vi "Initialize.vi"(8 "error in (no error)":errorcluster, 10 "Internal?":bool, 11 "Huber Settings In":T1) -> (0 "error out":errorcluster, 2 "Connection Error":bool, 3 "Huber Settings Out":T1)   [LabVIEW 2018, in "Huber Unistat 410 TCU.lvlib"]
uses:
  Huber Unistat 410 TCU.lvlib
  Huber Unistat 410 Settings.ctl
  <vilib>/Instr/_visa.llb/VISA Configure Serial Port (Instr).vi
panel:
  out "read string":string
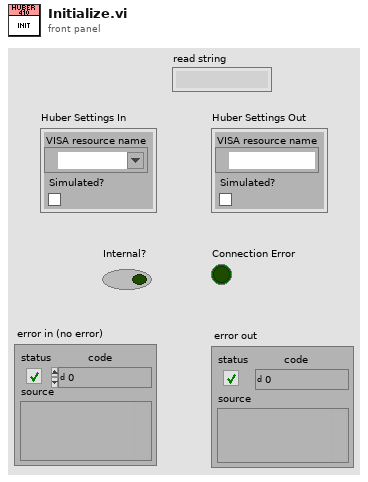
[diagram p1: front panel]
types:
  T1 = typedef "Huber Unistat 410 TCU.lvlib/Huber Unistat 410 Settings.ctl" = cluster{"VISA resource name":refnum<visa-resource-name>, "Simulated?":bool}
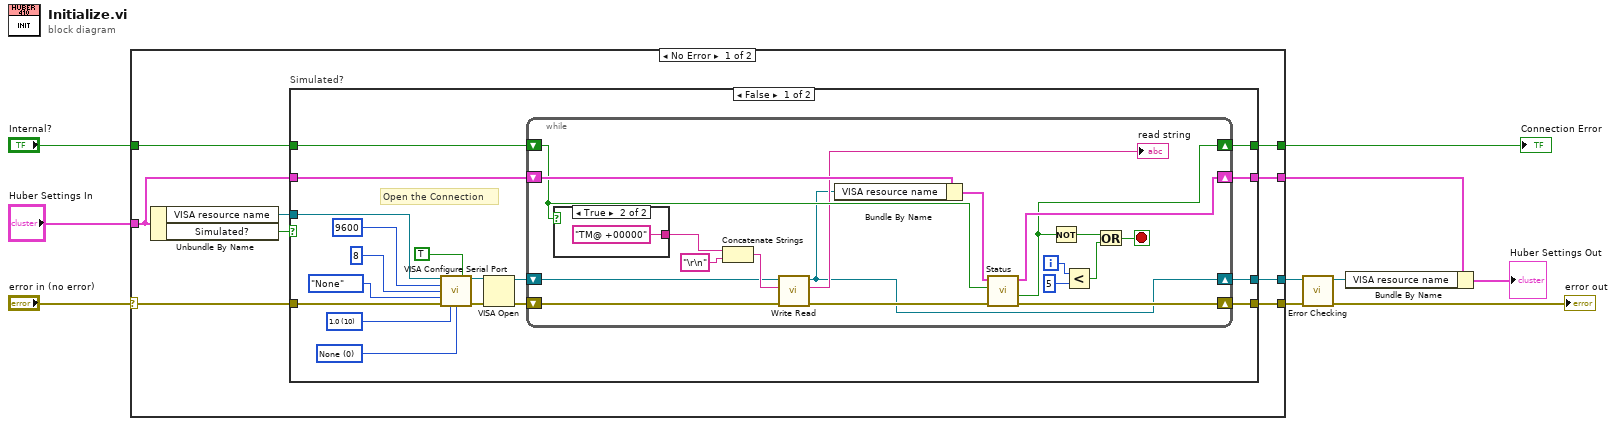
[diagram p0: block diagram]
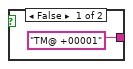
[diagram p2: hidden frame]
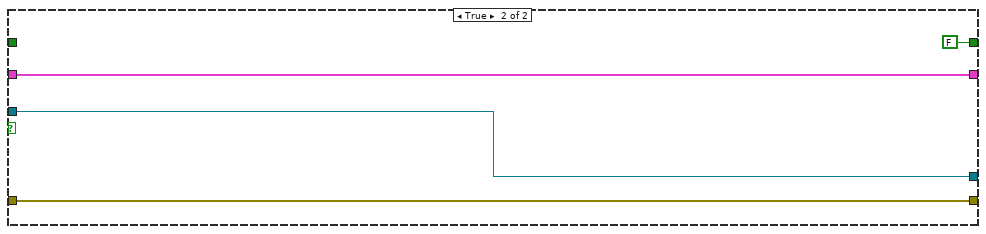
[diagram p3: hidden frame]
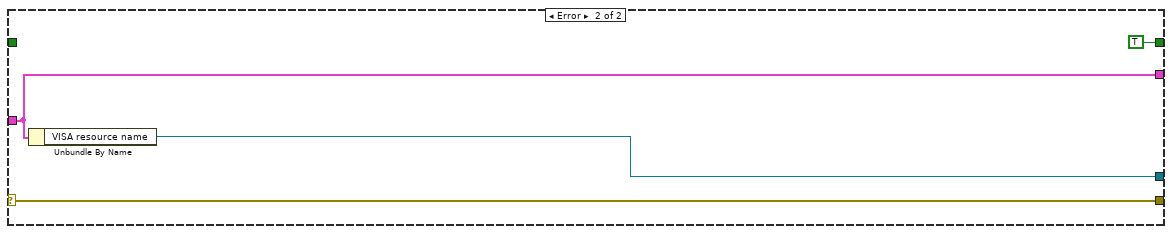
[diagram p4: hidden frame]
diagram:
  n1 = case shown="No Error" "error in (no error)" {
    selector: "error in (no error)" -> [w19 w66]
    tunnel: "Huber Settings In" -> [w13 w63]
    tunnel: [w18 w66] -> w8
    tunnel: [w16 w65] -> w9
    tunnel: [w14 TRUE] -> w4
    tunnel: [w12 w63] -> w3
    tunnel: "Internal?" -> [w11 _]
    frame No Error {
      n2 = Unbundle By Name(w13) -> ("VISA resource name"=w17:refnum<visa-resource-name>, "Simulated?"=w15:bool)
      n3 = case "Simulated?" shown="False" w15 {
        tunnel: w19 -> [w32 w62]
        tunnel: [w26 w62] -> w18
        tunnel: [w20 w61] -> w16
        tunnel: w17 -> [w31 w61]
        tunnel: [w28 FALSE] -> w14
        tunnel: w13 -> [w29 w59]
        tunnel: [w27 w59] -> w12
        tunnel: w11 -> [w25 _]
        frame False {
          w33 = u16 0 items=["None", "XON/XOFF", "RTS/CTS", "XON/XOFF & RTS/CTS", "DTR/DSR", "XON/XOFF & DTR/DSR"] ("flow control (0:none)")
          w34 = u16 10 items=["1.0"=10, "1.5"=15, "2.0"=20] ("stop bits (10: 1 bit)")
          # "Open the Connection"
          n4 = call-poly "VISA Configure Serial Port"("VISA resource name"=w31, "Enable Termination\nChar (T)"=TRUE ("Enable Termination\nChar (T)"), "baud rate (9600)"=u32 9600, "data bits (8)"=u16 8, "parity (0:none)"=enum16{"None", "Odd", "Even", "Mark", "Space"}."None", "error in (no error)"=w32, "stop bits (10: 1 bit)"=w34, "flow control (0:none)"=w33) -> ("VISA resource name out"=w23:refnum<visa-resource-name>, "error out"=w24:errorcluster)  [unwired: 6 in]
          n5 = VISA Open(error in (no error)=w24, VISA resource name=w23) -> (VISA resource name=w21:refnum<visa-resource-name>, error out=w22:errorcluster)  [unwired: 3 in]
          n6 = while {
            shift-right: [w53] -> w26
            shift-left: w22 -> [w40]
            shift-right: [w38] -> w20
            shift-left: w21 -> [w39]
            shift-right: [w54] -> w27
            shift-left: w29 -> [w56]
            shift-right: [w46] -> w28
            shift-left: w25 -> [w48]
            i -> [w45]
            stop <- w41 stop-if-true
            n7 = case shown="True" w48 {
              tunnel: ["TM@ +00001" "TM@ +00000"] -> w50
              frame False {
              }
              frame True {
              }
            }
            n8 = Concatenate Strings(w50, "\r\n" ("string")) -> (w51:string)
            n9 = call "Write Read.vi"("error in (no error)"=w40, "write string"=w51, "VISA Refnum in"=w39) -> ("error out"=w52:errorcluster, "read string"=→"read string":string, "VISA Refnum out"=w38:refnum<visa-resource-name>)  [unwired: 6 in]
            n10 = Bundle By Name(cluster=w56, "VISA resource name"=w38) -> (w55:T1)
            n11 = call "Status.vi"("error in (no error)"=w52, "Internal?"=w48, "Huber Settings In"=w55) -> ("error out"=w53:errorcluster, "Connection Error"=w46:bool, "Huber Settings Out"=w54:T1)  [unwired: 4 in, 2 out]
            n12 = Not(x=w46) -> (.not. x?=w43:bool)
            n13 = Less?(x=w45, y=5) -> (x < y?=w42:bool)
            n14 = Or(x=w43, y=w42) -> (x .or. y?=w41:bool)
          }
        }
        frame True {
        }
      }
    }
    frame Error {
      n15 = Unbundle By Name(w63) -> ("VISA resource name"=w65:refnum<visa-resource-name>)
    }
  }
  "Connection Error" <- w4
  n16 = call "Error Checking.vi"("error in (no error)"=w8, "VISA resource name"=w9) -> ("error out"=→"error out":errorcluster, "VISA resource name"=w6:refnum<visa-resource-name>)  [unwired: 7 in, 1 out]
  n17 = Bundle By Name(cluster=w3, "VISA resource name"=w6) -> (→"Huber Settings Out":T1)
